vi "ParseComic.vi"(7 "URL":string, 8 "error in (no error)":errorcluster, 11 "Issue":string) -> (0 "error out":errorcluster, 3 "comic":T1 {"Cover Price" format="$%.2g"})   [LabVIEW 2022 SP3]
uses:
  TypeDefs/Comic.ctl
  TypeDefs/Character.ctl
  TypeDefs/Creator.ctl
  TypeDefs/Variant.ctl
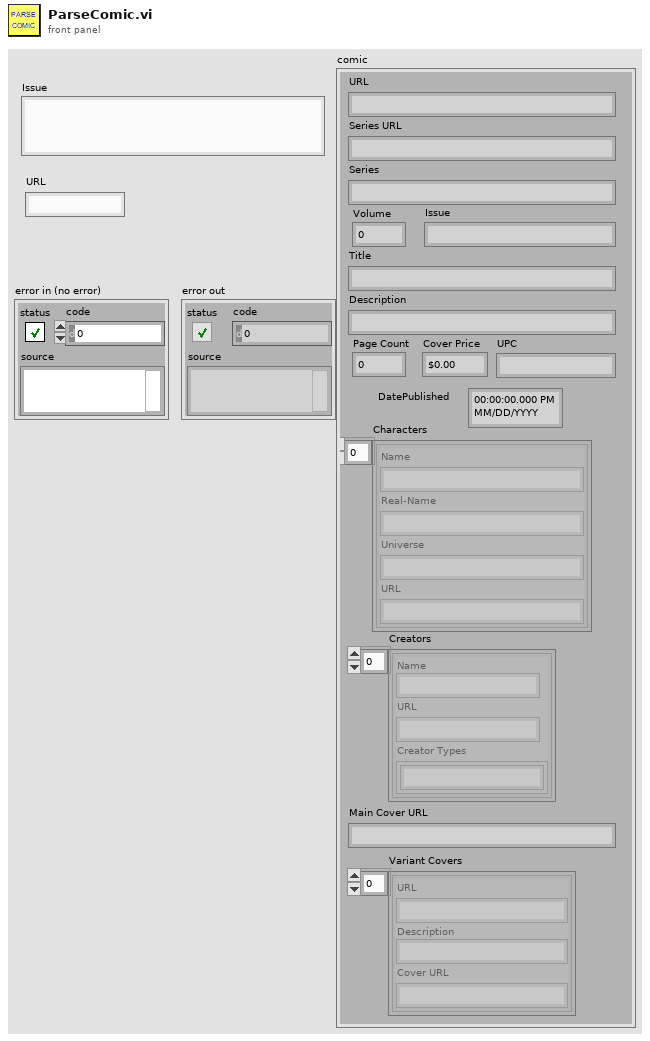
[diagram p1: front panel]
types:
  T1 = typedef "Comic.ctl" = cluster{"URL":string, "Series URL":string, "Series":string, "Volume":i32, "Issue":string, "Title":string, "Description":string, "Page Count":i32, "Cover Price":dbl, "UPC":string, "Characters":T2[], "Creators":T3[], "Main Cover URL":string, "Variant Covers":T4[], "DatePublished":timestamp}
  T2 = typedef "Character.ctl" = cluster{"Name":string, "Real-Name":string, "Universe":string, "URL":string}
  T3 = typedef "Creator.ctl" = cluster{"Name":string, "URL":string, "Creator Types":string[]}
  T4 = typedef "Variant.ctl" = cluster{"URL":string, "Description":string, "Cover URL":string}
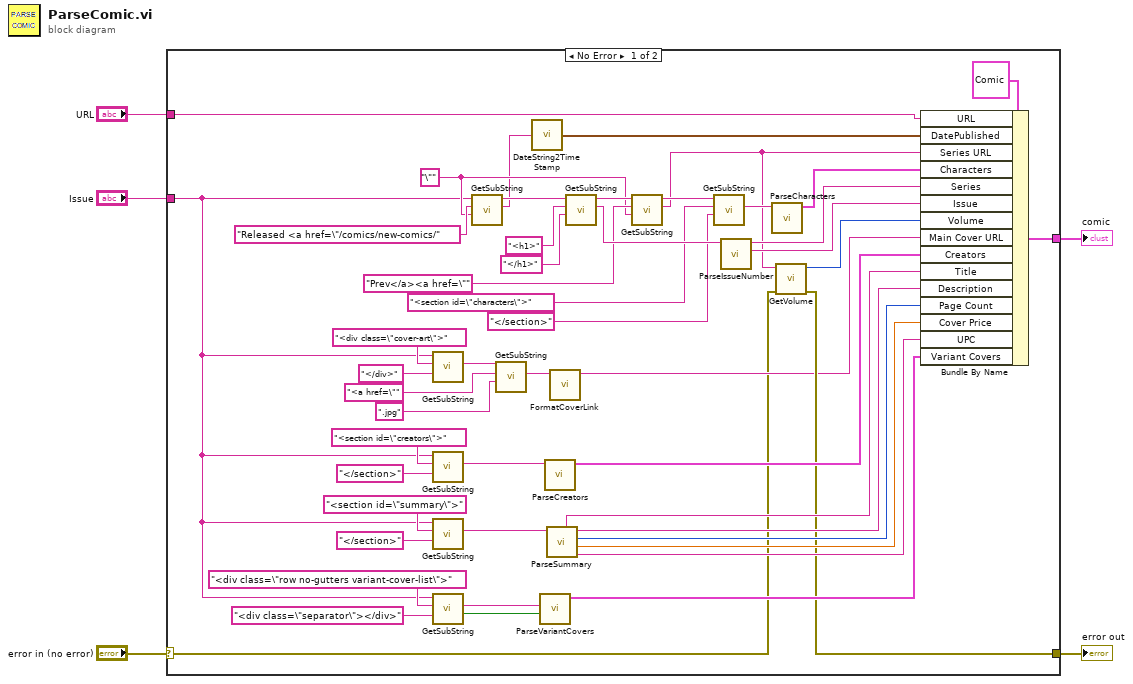
[diagram p0: block diagram]
diagram:
  n1 = case shown="No Error" "error in (no error)" {
    selector: "error in (no error)" -> [w6 w55]
    tunnel: [w31 _] -> w5
    tunnel: "URL" -> [w26 _]
    tunnel: "Issue" -> [w15 _]
    tunnel: [w11 w55] -> w2
    frame No Error {
      w47 = "\"" ("End Search")
      n2 = call "GetSubString.vi"("End Search"="</div>", "Start Search"="<div class=\"cover-art\">", "String In"=w15) -> ("Match"=w39:string)  [unwired: 6 in, 2 out]
      n3 = call "GetSubString.vi"("End Search"="</section>", "Start Search"="<section id=\"creators\">", "String In"=w15) -> ("Match"=w28:string)  [unwired: 6 in, 2 out]
      n4 = call "GetSubString.vi"("End Search"="</section>", "Start Search"="<section id=\"summary\">", "String In"=w15) -> ("Match"=w23:string)  [unwired: 6 in, 2 out]
      n5 = call "GetSubString.vi"("End Search"="<div class=\"separator\"></div>", "Start Search"="<div class=\"row no-gutters variant-cover-list\">", "String In"=w15) -> ("Not Found?"=w13:bool, "Match"=w14:string)  [unwired: 6 in, 1 out]
      n6 = call "GetSubString.vi"("End Search"=w47, "Start Search"="Released <a href=\"/comics/new-comics/", "String In"=w15) -> ("Match"=w42:string, "Following String Out"=w53:string)  [unwired: 6 in, 1 out]
      n7 = call "GetSubString.vi"("End Search"=".jpg", "Start Search"="<a href=\"" ("End Search"), "String In"=w39) -> ("Match"=w32:string)  [unwired: 6 in, 2 out]
      n8 = call "DateString2TimeStamp.vi"("DateString(YYYY/MM/DD)"=w42) -> ("time stamp"=w35:timestamp)  [unwired: 4 in]
      n9 = call "ParseVariantCovers.vi"("Covers Not Found?"=w13, "CoversSubSection"=w14) -> ("VariantCovers"=w12:T4[])  [unwired: 9 in]
      n10 = call "ParseCreators.vi"("Raw HTML"=w28) -> ("Creators"=w27:T3[])  [unwired: 10 in]
      n11 = call "ParseSummary.vi"("Section"=w23) -> ("UPC"=w18:string, "Price"=w19:dbl, "Pages"=w20:i32, "Description"=w21:string, "Title"=w22:string)  [unwired: 6 in]
      n12 = call "FormatCoverLink.vi"("Cover Link"=w32) -> ("result string"=w9:string)  [unwired: 10 in]
      n13 = call "GetSubString.vi"("End Search"="</h1>", "Start Search"="<h1>", "String In"=w53) -> ("Match"=w50:string, "Following String Out"=w49:string)  [unwired: 6 in, 1 out]
      n14 = call "GetSubString.vi"("End Search"=w47, "Start Search"="Prev</a><a href=\"", "String In"=w49) -> ("Match"=w7:string, "Following String Out"=w45:string)  [unwired: 6 in, 1 out]
      n15 = call "GetSubString.vi"("End Search"="</section>", "Start Search"="<section id=\"characters\">", "String In"=w45) -> ("Match"=w43:string)  [unwired: 6 in, 2 out]
      n16 = call "ParseIssueNumber.vi"("String In"=w50) -> ("Issue"=w33:string, "Series"=w10:string)  [unwired: 9 in]
      n17 = call "ParseCharacters.vi"("TextIn"=w43) -> ("Characters"=w34:T2[])  [unwired: 10 in]
      n18 = call "GetVolume.vi"("error in (no error)"=w6, "SeriesURL"=w7) -> ("error out"=w11:errorcluster, "Volume"=w8:i32)  [unwired: 8 in]
      n19 = Bundle By Name(cluster=T1 {"URL"="", "Series URL"="", "Series"="", "Volume"=0, "Issue"="", "Title"="", "Description"="", "Page Count"=0, "Cover Price"=0.0, "UPC"="", "Characters"=[], "Creators"=[], "Main Cover URL"="", "Variant Covers"=[], "DatePublished"=timestamp(0 s since 1904-01-01)} ("Comic"), "URL"=w26, "DatePublished"=w35, "Series URL"=w7, "Characters"=w34, "Series"=w10, "Issue"=w33, "Volume"=w8, "Main Cover URL"=w9, "Creators"=w27, "Title"=w22, "Description"=w21, "Page Count"=w20, "Cover Price"=w19, "UPC"=w18, "Variant Covers"=w12) -> (w31:T1)
    }
    frame Error {
    }
  }
  "comic" <- w5
  "error out" <- w2
